vi "Populate Menu.vi"(8 "error in (no error)":errorcluster, 9 "Coords":T1, 10 "MenuRef":refnum<k9>, 11 "Process Builder View in":refnum<class "Process Builder View.lvclass">) -> (0 "error out":errorcluster, 2 "Discard?":bool, 3 "Process Builder View out":refnum<class "Process Builder View.lvclass">)   [LabVIEW 2019, in "Process Builder View.lvclass"]
uses:
  <vilib>/gpm_packages/@cs/Car-wash/Source/Process Builder View/Process Builder View.lvclass
  C:/Program Files/National Instruments/LabVIEW 2019/vi.lib/gpm_packages/@cs/Test-executive-builder/Source/Test Executive Builder View/Test Executive Builder View/Test Executive Builder View.lvclass
  <vilib>/Utility/miscctls.llb/LVPoint32TypeDef.ctl
  <vilib>/gpm_packages/@cs/Test-executive-builder/Source/Test Executive Builder View/Test Executive Builder View/Test Executive Builder View.lvclass/Test Executive Builder View.ctl
  <vilib>/gpm_packages/@cs/Test-executive-builder/Source/Test Executive Builder View/Tree Click Interpreter/Tree Click Interpreter.lvclass
  <vilib>/gpm_packages/@cs/Test-executive-builder/Source/Test Executive Builder View/Test Executive Builder View/Test Executive Builder View.lvclass
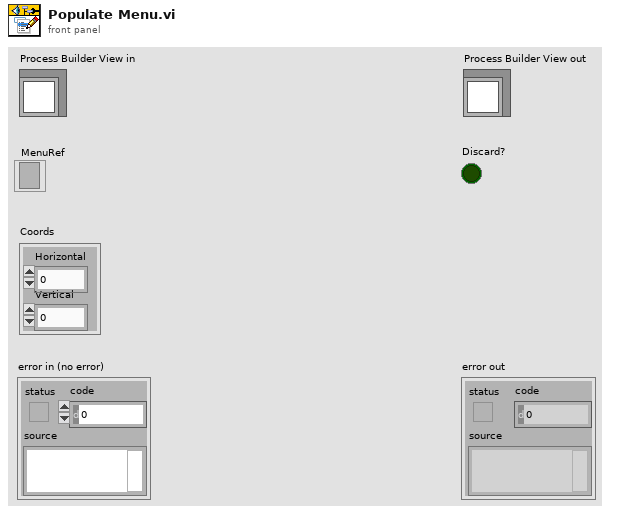
[diagram p1: front panel]
types:
  T1 = typedef "LVPoint32TypeDef.ctl" = cluster{"Horizontal":i32, "Vertical":i32}
  T2 = typedef "Relative Click Location.ctl" = enum16{"Unknown Location", "Below Element", "On Element", "Above Element"}
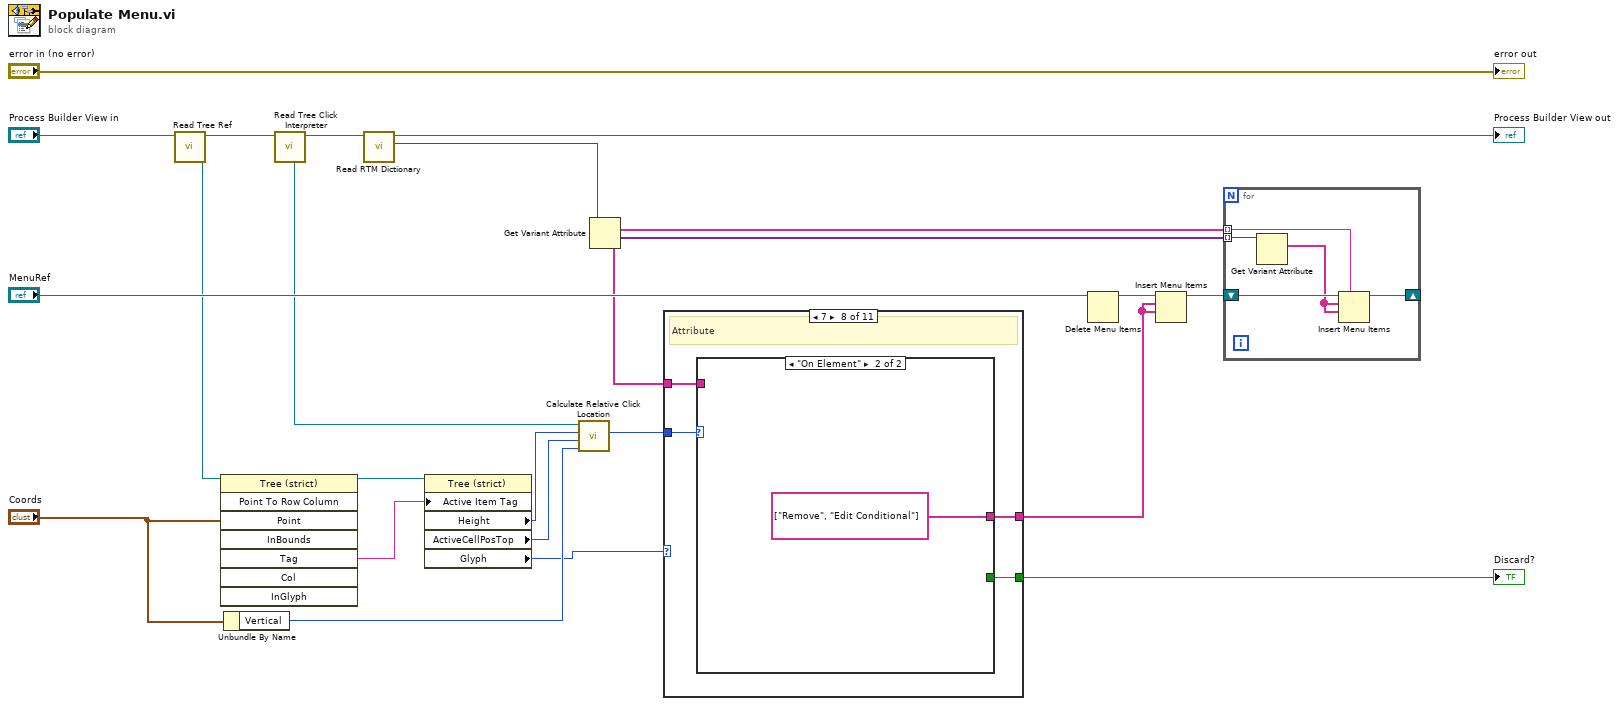
[diagram p0: block diagram]
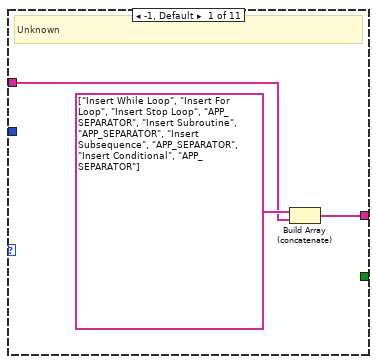
[diagram p2: hidden frame]
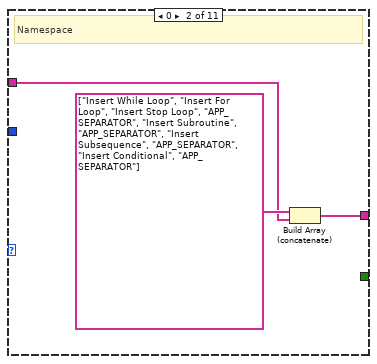
[diagram p3: hidden frame]
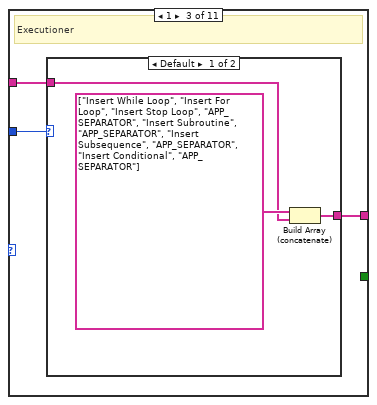
[diagram p4: hidden frame]
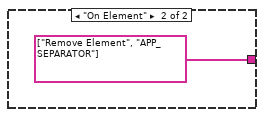
[diagram p5: hidden frame]
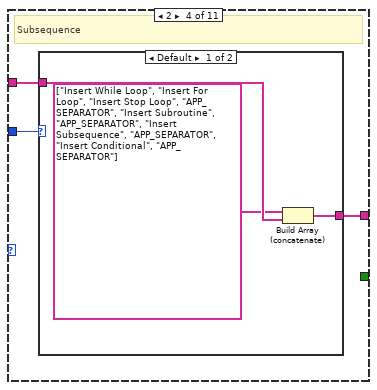
[diagram p6: hidden frame]
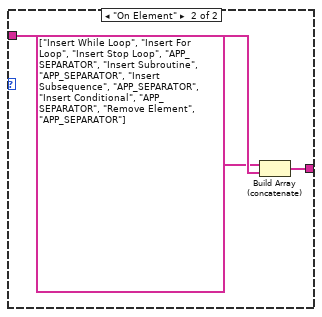
[diagram p7: hidden frame]
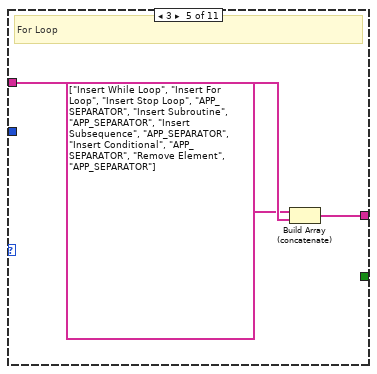
[diagram p8: hidden frame]
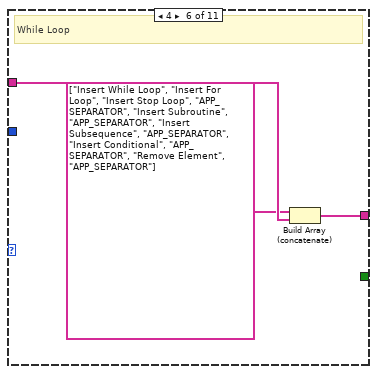
[diagram p9: hidden frame]
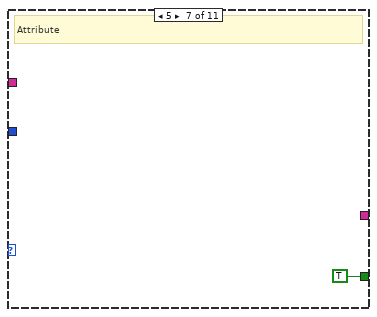
[diagram p10: hidden frame]
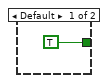
[diagram p11: hidden frame]
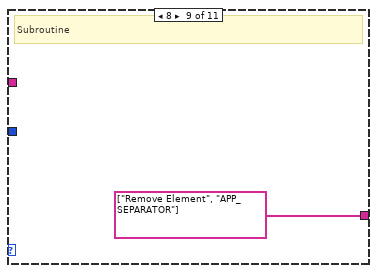
[diagram p12: hidden frame]
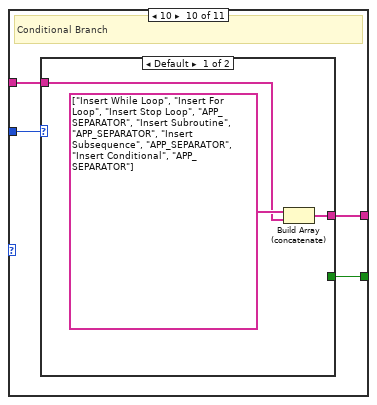
[diagram p13: hidden frame]
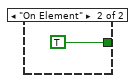
[diagram p14: hidden frame]
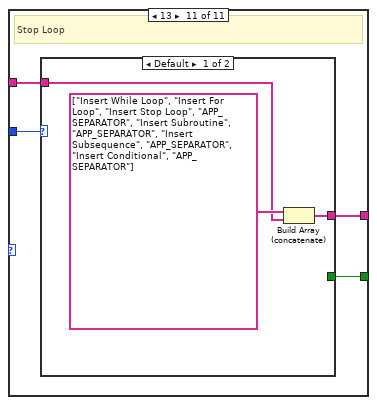
[diagram p15: hidden frame]
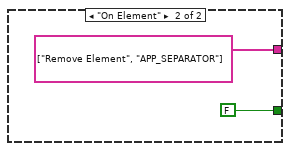
[diagram p16: hidden frame]
diagram:
  n1 = call <vilib>:"Read Tree Ref.vi"("Test Executive Builder View in"="Process Builder View in") -> ("Tree Ref"=w14:refnum<vi>, "Test Executive Builder View out"=w18:refnum<class "Process Builder View.lvclass">)  [unwired: 9 in]
  n2 = invoke class="Tree (strict)" method="Point To Row Column"(reference=w14, "Point"="Coords") -> (reference out=w13:refnum<vi>, "Tag"=w12:string)  [unwired: 6 in, 6 out]
  n3 = Unbundle By Name("Coords") -> ("Vertical"=w8:i32)
  n4 = call <vilib>:"Read Tree Click Interpreter.vi"("Test Executive Builder View in"=w18) -> ("Test Executive Builder View out"=w16:refnum<class "Process Builder View.lvclass">, "Tree Click Interpreter"=w15:refnum<class "Tree Click Interpreter.lvclass">)  [unwired: 9 in]
  n5 = call <vilib>:"Read RTM Dictionary.vi"("Test Executive Builder View in"=w16) -> ("RTM Dictionary"=w7:variant, "Test Executive Builder View out"=→"Process Builder View out":refnum<class "Process Builder View.lvclass">)  [unwired: 9 in]
  n6 = property class="Tree (strict)"(reference=w13, "Active Item Tag"=w12) -> ("Height"=w11:i32, "ActiveCellPosTop"=w10:i32, "Glyph"=w4:i32)  [unwired: 1 in, 2 out]
  n7 = call-dynamic "Calculate Relative Click Location.vi"("Click Vertical Position"=w8, "Cell Top Position"=w10, "Cell Height"=w11, "Tree Click Interpreter in"=w15) -> ("Relative Click Location"=w3:T2)  [unwired: 6 in, 1 out]
  n8 = Get Variant Attribute(Variant=w7) -> (names=w2:string[], values=w6:variant[])  [unwired: 3 in, 2 out]
  n9 = case shown="7" w4 {
    tunnel: [w25 w28 w32 w39 w48 w51 _ w53 string[] ["Remove Element", "APP_SEPARATOR"] w61 w69] -> w21
    tunnel: w3 -> [_ _ w30 w37 _ _ _ w54 _ w62 w70]
    tunnel: w2 -> [w24 w27 w31 w38 w47 w50 _ w55 _ w63 w71]
    tunnel: [_ _ _ _ _ _ TRUE w56 _ w60 w68] -> w1
    frame -1, Default {
      # "Unknown"
      n10 = Build Array (concatenate)(string[] ["Insert While Loop", "Insert For Loop", "Insert Stop Loop", "APP_SEPARATOR", "Insert Subroutine", "APP_SEPARATOR", "Insert Subsequence", "APP_SEPARATOR", "Insert Conditional", "APP_SEPARATOR"], w24) -> (w25:string[])
    }
    frame 0 {
      # "Namespace"
      n11 = Build Array (concatenate)(string[] ["Insert While Loop", "Insert For Loop", "Insert Stop Loop", "APP_SEPARATOR", "Insert Subroutine", "APP_SEPARATOR", "Insert Subsequence", "APP_SEPARATOR", "Insert Conditional", "APP_SEPARATOR"], w27) -> (w28:string[])
    }
    frame 1 {
      # "Executioner"
      n12 = case shown="Default" w30 {
        tunnel: [w34 string[] ["Remove Element", "APP_SEPARATOR"]] -> w32
        tunnel: w31 -> [w33 _]
        frame Default {
          n13 = Build Array (concatenate)(string[] ["Insert While Loop", "Insert For Loop", "Insert Stop Loop", "APP_SEPARATOR", "Insert Subroutine", "APP_SEPARATOR", "Insert Subsequence", "APP_SEPARATOR", "Insert Conditional", "APP_SEPARATOR"], w33) -> (w34:string[])
        }
        frame "On Element" {
        }
      }
    }
    frame 2 {
      # "Subsequence"
      n14 = case shown="Default" w37 {
        tunnel: [w42 w45] -> w39
        tunnel: w38 -> [w41 w44]
        frame Default {
          n15 = Build Array (concatenate)(string[] ["Insert While Loop", "Insert For Loop", "Insert Stop Loop", "APP_SEPARATOR", "Insert Subroutine", "APP_SEPARATOR", "Insert Subsequence", "APP_SEPARATOR", "Insert Conditional", "APP_SEPARATOR"], w41) -> (w42:string[])
        }
        frame "On Element" {
          n16 = Build Array (concatenate)(string[] ["Insert While Loop", "Insert For Loop", "Insert Stop Loop", "APP_SEPARATOR", "Insert Subroutine", "APP_SEPARATOR", "Insert Subsequence", "APP_SEPARATOR", "Insert Conditional", "APP_SEPARATOR", "Remove Element", "APP_SEPARATOR"], w44) -> (w45:string[])
        }
      }
    }
    frame 3 {
      # "For Loop"
      n17 = Build Array (concatenate)(string[] ["Insert While Loop", "Insert For Loop", "Insert Stop Loop", "APP_SEPARATOR", "Insert Subroutine", "APP_SEPARATOR", "Insert Subsequence", "APP_SEPARATOR", "Insert Conditional", "APP_SEPARATOR", "Remove Element", "APP_SEPARATOR"], w47) -> (w48:string[])
    }
    frame 4 {
      # "While Loop"
      n18 = Build Array (concatenate)(string[] ["Insert While Loop", "Insert For Loop", "Insert Stop Loop", "APP_SEPARATOR", "Insert Subroutine", "APP_SEPARATOR", "Insert Subsequence", "APP_SEPARATOR", "Insert Conditional", "APP_SEPARATOR", "Remove Element", "APP_SEPARATOR"], w50) -> (w51:string[])
    }
    frame 5 {
      # "Attribute"
    }
    frame 7 {
      # "Attribute"
      n19 = case shown="\"On Element\"" w54 {
        tunnel: [TRUE _] -> w56
        tunnel: w55 -> [_ _]
        tunnel: [_ string[] ["Remove", "Edit Conditional"]] -> w53
        frame Default {
        }
        frame "On Element" {
        }
      }
    }
    frame 8 {
      # "Subroutine"
    }
    frame 10 {
      # "Conditional Branch"
      n20 = case shown="Default" w62 {
        tunnel: [w65 _] -> w61
        tunnel: w63 -> [w64 _]
        tunnel: [_ TRUE] -> w60
        frame Default {
          n21 = Build Array (concatenate)(string[] ["Insert While Loop", "Insert For Loop", "Insert Stop Loop", "APP_SEPARATOR", "Insert Subroutine", "APP_SEPARATOR", "Insert Subsequence", "APP_SEPARATOR", "Insert Conditional", "APP_SEPARATOR"], w64) -> (w65:string[])
        }
        frame "On Element" {
        }
      }
    }
    frame 13 {
      # "Stop Loop"
      n22 = case shown="Default" w70 {
        tunnel: [w73 string[] ["Remove Element", "APP_SEPARATOR"]] -> w69
        tunnel: w71 -> [w72 _]
        tunnel: [_ FALSE] -> w68
        frame Default {
          n23 = Build Array (concatenate)(string[] ["Insert While Loop", "Insert For Loop", "Insert Stop Loop", "APP_SEPARATOR", "Insert Subroutine", "APP_SEPARATOR", "Insert Subsequence", "APP_SEPARATOR", "Insert Conditional", "APP_SEPARATOR"], w72) -> (w73:string[])
        }
        frame "On Element" {
        }
      }
    }
  }
  "Discard?" <- w1
  n24 = Delete Menu Items(9:"MenuRef") -> (3:w22:refnum<k9>)  [unwired: 3 in, 1 out]
  n25 = Insert Menu Items(7:w21, 8:w21, 9:w22) -> (3:w5:refnum<k9>)  [unwired: 3 in, 2 out]
  n26 = for {
    tunnel: w2 -> [w78] mode=indexing
    tunnel: w6 -> [w81] mode=indexing
    shift-right: [w79] -> _
    shift-left: w5 -> [w80]
    n27 = Get Variant Attribute(Variant=w81) -> (names=w77:string[])  [unwired: 3 in, 3 out]
    n28 = Insert Menu Items(5:w78, 7:w77, 8:w77, 9:w80) -> (3:w79:refnum<k9>)  [unwired: 2 in, 2 out]
  }
  "error out" <- "error in (no error)"
